vi "main.vi"(11 "launched":refnum<notifier>) -> ()   [LabVIEW 2020]
uses:
  _controls/save_options.ctl
  _controls/checkbox.ctl
  _controls/button.rec.ctl
  camera/camera.lvclass
  <vilib>/Utility/sysdir.llb/System Directory Type.ctl
  _controls/state.ctl
  _controls/DLL.state.ctl
  fb840919-9eb0-46b6-9bb3-d477681bf041.vi
  1d8e8226-7041-439d-8714-8787373e7ba9.vi
  8fbd63eb-6e1f-4c86-bab6-28681c6e18d2.vi
  86724869-5739-4cd7-b902-c7d6e6aa67a1.vi
  55541a10-fe72-4f23-aa32-8552e1fca114.vi
  782ab28e-0829-4b0f-8f82-3ba71064f937.vi
  21b5fd2b-e315-48a8-934d-9fb4121eccaa.vi
  c147b8e2-e97a-4fb6-9f9b-10b3bfa32c03.vi
  d040b064-8120-4bee-ba75-bc9a352b41e4.vi
  f030127b-7363-4f40-9caf-aa7af2fa5467.vi
  a77384f8-0254-4858-83b2-e693f57fe95f.vi
  c0d7e7e1-aa2c-47d6-a73c-058c71d33236.vi
  eef2a813-7c02-4df4-9d88-e87a40ecc536.vi
  96ad7128-a59b-4646-90f0-c775a03dfb8e.vi
  094a7fb3-58c3-48c3-896b-6fa17c1e0ca1.vi
  06917477-7661-483e-91a3-5a2f461782c2.vi
  e584de4e-bacd-4d82-b84f-7ed3eb6609c4.vi
  8bc19d28-31cb-4a7e-a618-0f8835e17850.vi
  3f5928e4-84ec-4848-af44-f012adbf1426.vi
  56f6947d-e80c-43c6-ba91-a3ae61841505.vi
  SubVI/img.Percentile.vi
  SubVI/pix.sgl.CalcPercentiles.sgl.vi
  <vilib>/Utility/file.llb/Application Directory.vi
  <vilib>/Utility/config.llb/Open Config Data.vi
  <vilib>/Utility/config.llb/Read Key.vi
  <vilib>/Utility/config.llb/Read Key (Boolean).vi
  <vilib>/Utility/config.llb/Write Key.vi
  <vilib>/Utility/config.llb/Write Key (Boolean).vi
  SubVI/error.RebrandExistingError.vi
  <vilib>/Utility/config.llb/Close Config Data.vi
  <vilib>/Utility/config.llb/Read Key (String).vi
  <vilib>/Utility/config.llb/Write Key (String).vi
  <vilib>/Utility/config.llb/Read Key (U32).vi
  <vilib>/Utility/config.llb/Write Key (U32).vi
  <vilib>/Utility/config.llb/Read Key (Double).vi
  <vilib>/Utility/config.llb/Write Key (Double).vi
  <vilib>/Utility/config.llb/Read Key (I32).vi
  <vilib>/Utility/config.llb/Write Key (I32).vi
  <vilib>/Utility/config.llb/Read Key (Path).vi
  <vilib>/Utility/config.llb/Write Key (Path).vi
  _accessors/DVR.vars.Read.vi
  SubVI/acq.Filename.vi
  <vilib>/Utility/libraryn.llb/Check if File or Folder Exists.vi
  SubVI/file.IsValid.vi
  SubVI/pix.sgl.CalcPercentiles.vi
  36df9122-e4f2-4645-ba20-61a7cd497c98.vi
panel:
  out "msg":string="Closing Program..."
  in  "fit":bool
  in  "minus":bool
  in  "plus":bool
  in  "FPS (For PL only)":dbl=30.0 min=5.0 max=100.0 step=5.0
  in  "array":bool
  out "recording":string="Recording..."
  in  "Exposure":u32=30 min=5 max=1000 step=5
  out "Image":T1(plugin-control)
  out "sub#":string
  in  "rightTab":enum32{"Acquisition", "Settings"}(tab)
  in  "state":T2(radio)=enum."Video"
  in  "Same?":T3
  in  "#":u32
  in  "video":T4 caption="Save Video"
  in  "histogram.enable":bool caption="Enable"
  in  "# bins":i32=20 caption="Bins bins" min=5 max=50 step=1
  in  "save.op":T5 caption="Save Option"
  in  "base_folder":cluster{"folder":path, "Tif":bool, "Jpg":bool}={"folder"=path "", "Tif"=TRUE, "Jpg"=TRUE}
  in  "Gain":enum16{"Low", "High"}(ring)
  out "histogram":cluster{"Axis":dbl[], "Histogram":i32[]}(graph)
  in  "Acquisitions":u64=5 min=1 max=500 step=1
  in  "Module Name":string="Module"
  in  "Min Value":i32=3 min=0 max=65535
  in  "Max Value":i32=97 min=1 max=65535
  in  "mapping":u32(ring)=16 items=["Default"=10, "Most Significant Bits"=11, "Full Dynamic"=12, "Downshift"=13, "Given Range"=14, "90% Dynamic"=15, "Given Percent Range"=16]
  out "progress":u8(slide) scale=0.0..10.0
  # "ACQ PARAMETERS"
  # "CAMERA"
  # "ACQUISITION"
  # "SAVE"
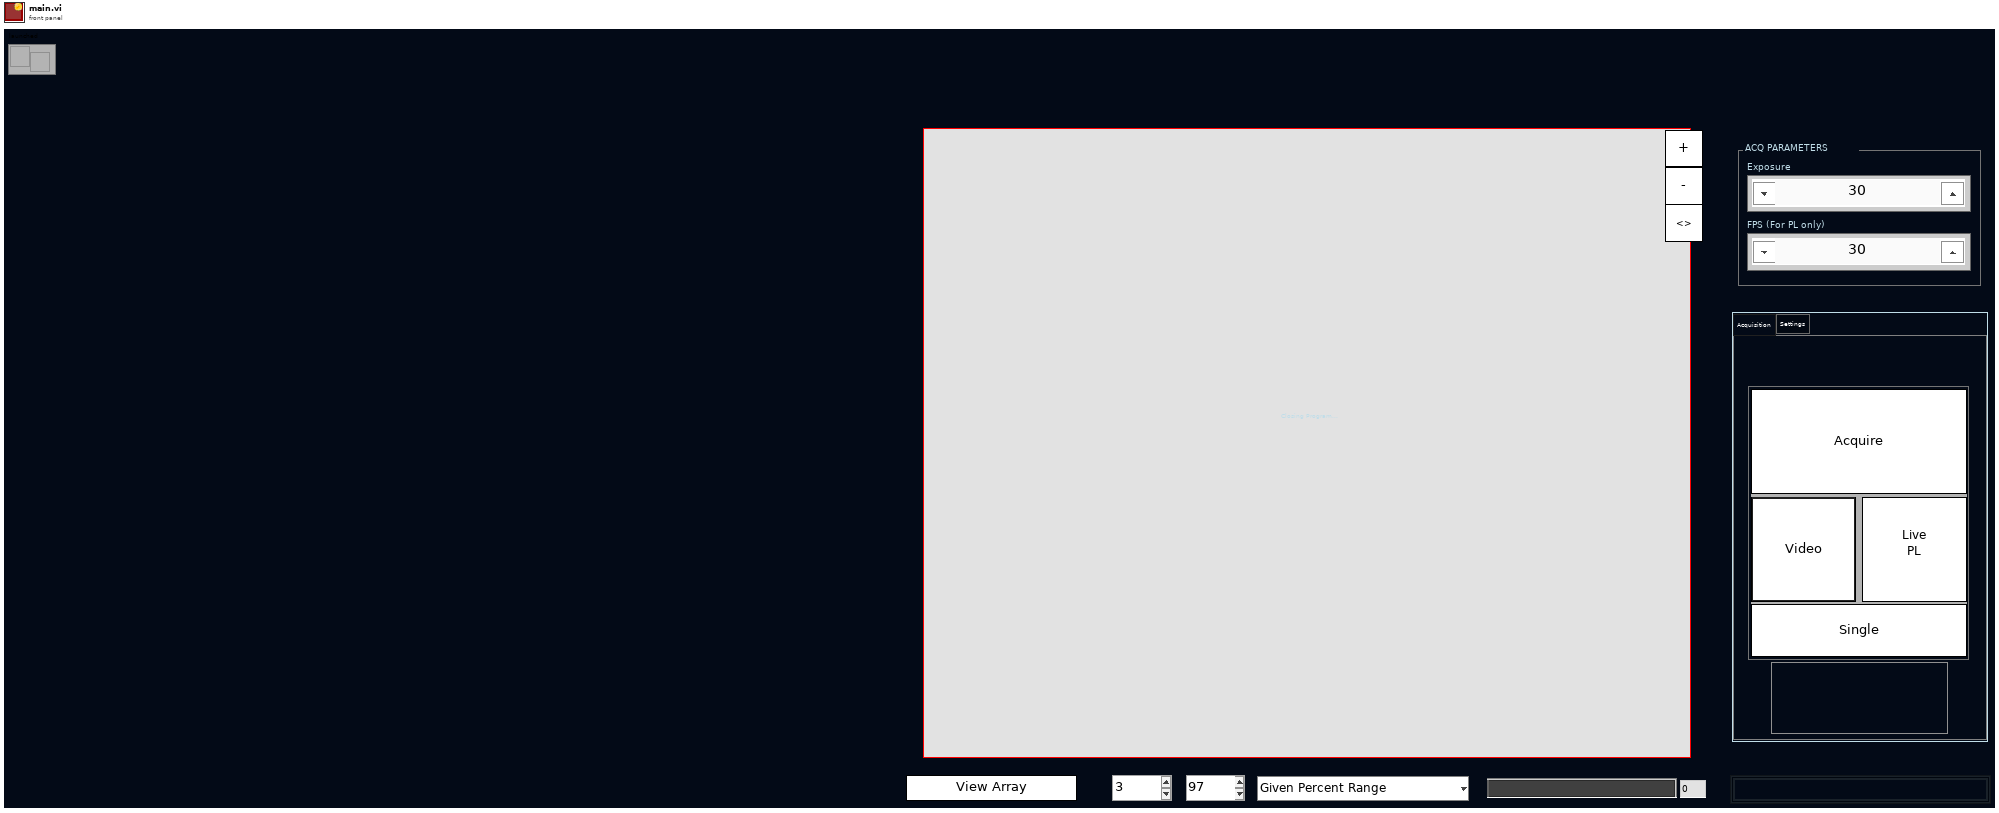
[diagram p1: front panel]
types:
  T1 = typedef "IMAQ Image.ctl" = refnum<image>
  T2 = enum32{"Switch", "Single", "Video", "Live", "none"}
  T3 = typedef "checkbox.ctl" = bool
  T4 = typedef "button.rec.ctl" = bool
  T5 = typedef "save_options.ctl" = enum16{"Light", "Full"}
  T6 = typedef "data.ctl" = cluster{"cam":refnum<class "camera.lvclass">, "ref":T7, "Q":cluster{"acq":cluster{"img1":refnum<queue>}, "display":cluster{"image":refnum<queue>}}, "timing":cluster{"state":refnum<queue>, "closeLoop":refnum<notifier>, "stop":refnum<k4>}, "vars":refnum<data-value>}
  T7 = typedef "data.ref.ctl" = cluster{"This VI":refnum<vi>, "rightPanel":refnum<vi>, "btn":cluster{"action":cluster{"Single":refnum<vi>, "Live":refnum<vi>, "Switch":refnum<vi>, "Video":refnum<vi>}, "Close":refnum<vi>}, "control":cluster{"#":refnum<vi>, "sub#":refnum<vi>, "auto_exp":refnum<vi>, "# Acq":refnum<vi>, "recording":refnum<vi>}, "graph":cluster{"img":T1, "avi":T1}}
  T8 = enum8{"Enabled", "Disabled", "Disabled and Grayed Out"}
  T9 = typedef "state.ctl" = enum16{"-", "single", "video", "livePL", "PL"}
  T10 = cluster{"Left":i32, "Top":i32, "Right":i32, "Bottom":i32}
  T11 = typedef "Image Type" = u32
  T12 = typedef "System Directory Type.ctl" = i32
  T13 = typedef "DLL.state.ctl" = u16
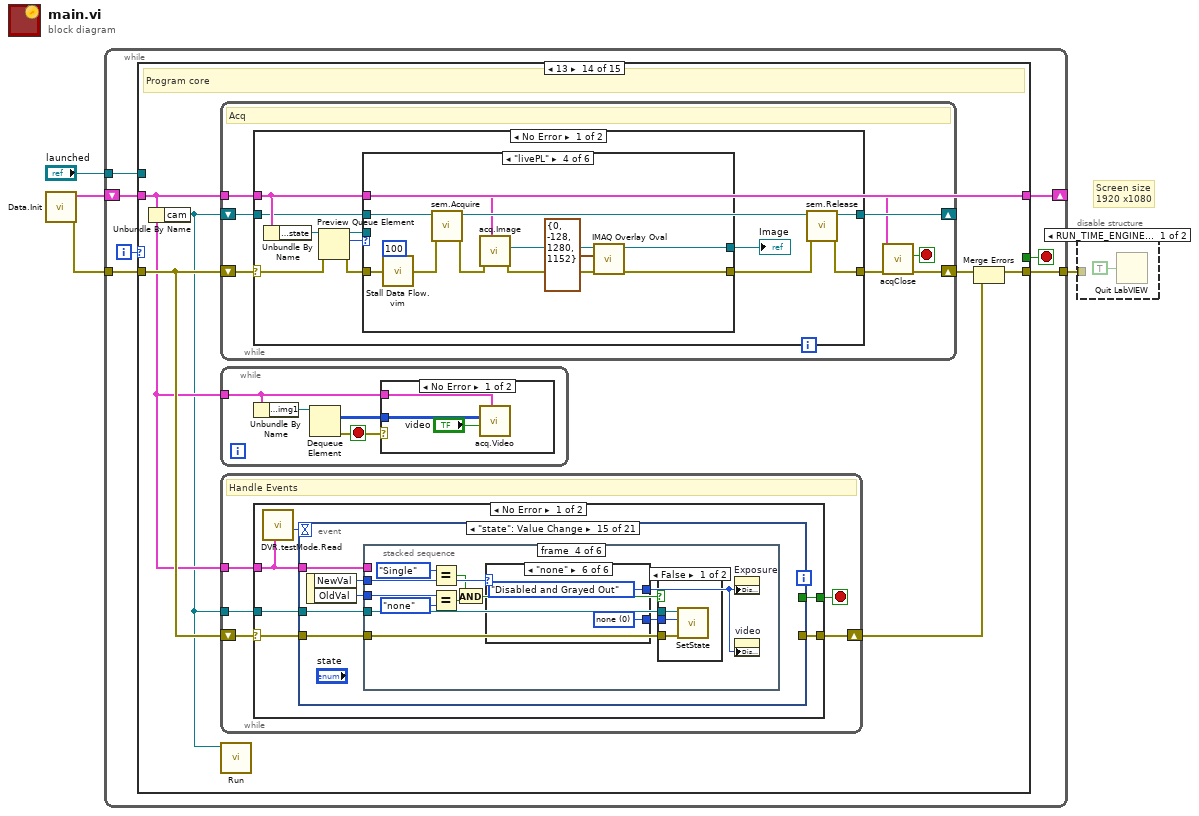
[diagram p0: block diagram]
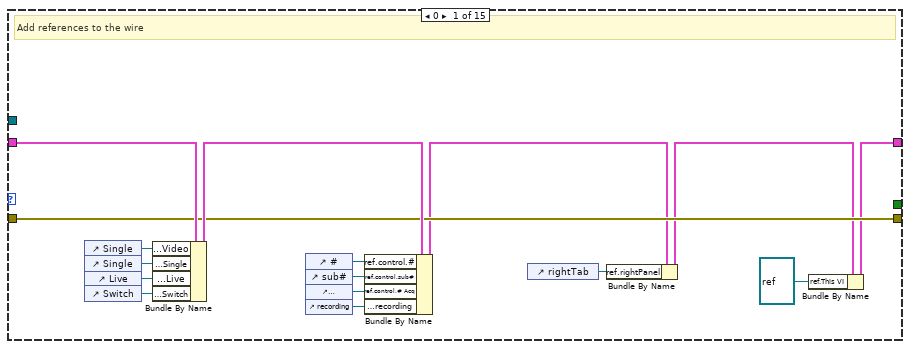
[diagram p2: hidden frame]
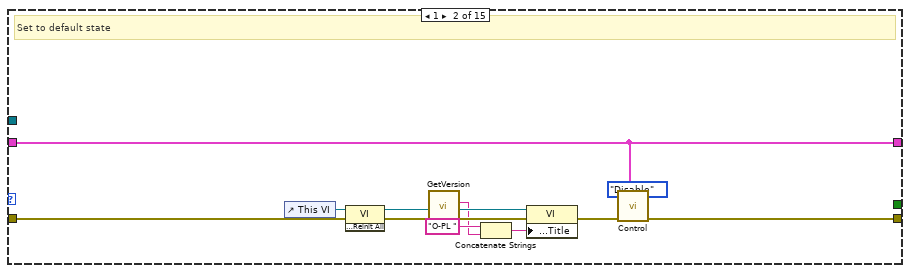
[diagram p3: hidden frame]
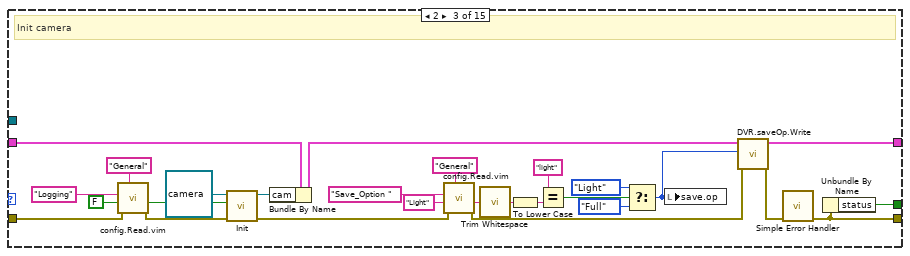
[diagram p4: hidden frame]
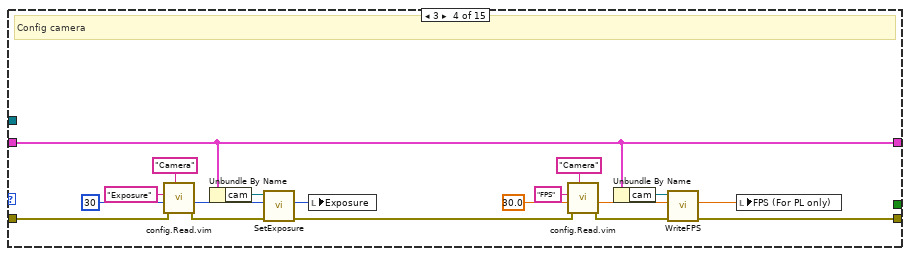
[diagram p5: hidden frame]
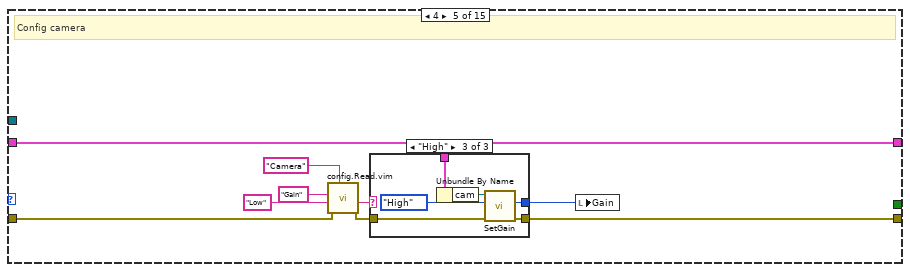
[diagram p6: hidden frame]
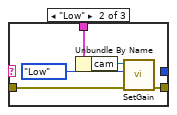
[diagram p8: hidden frame]
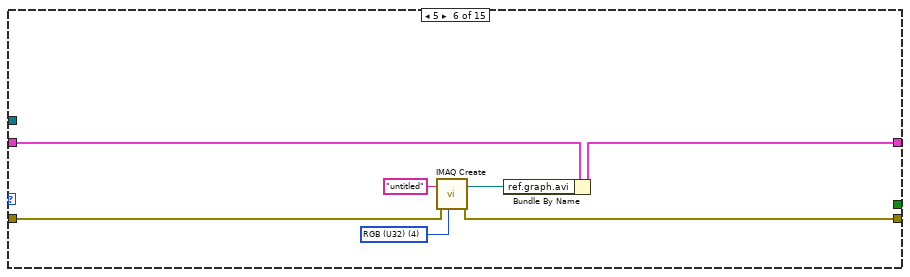
[diagram p9: hidden frame]
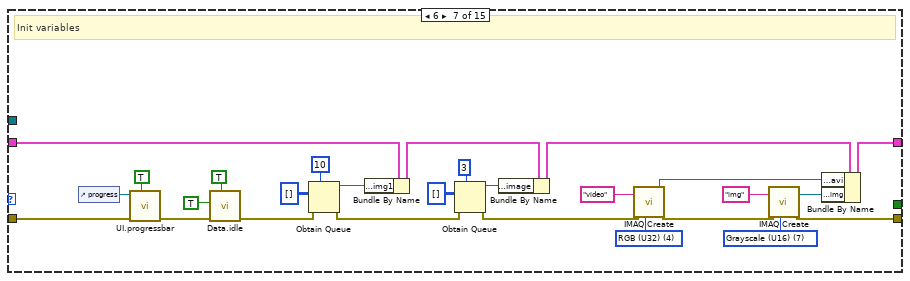
[diagram p10: hidden frame]
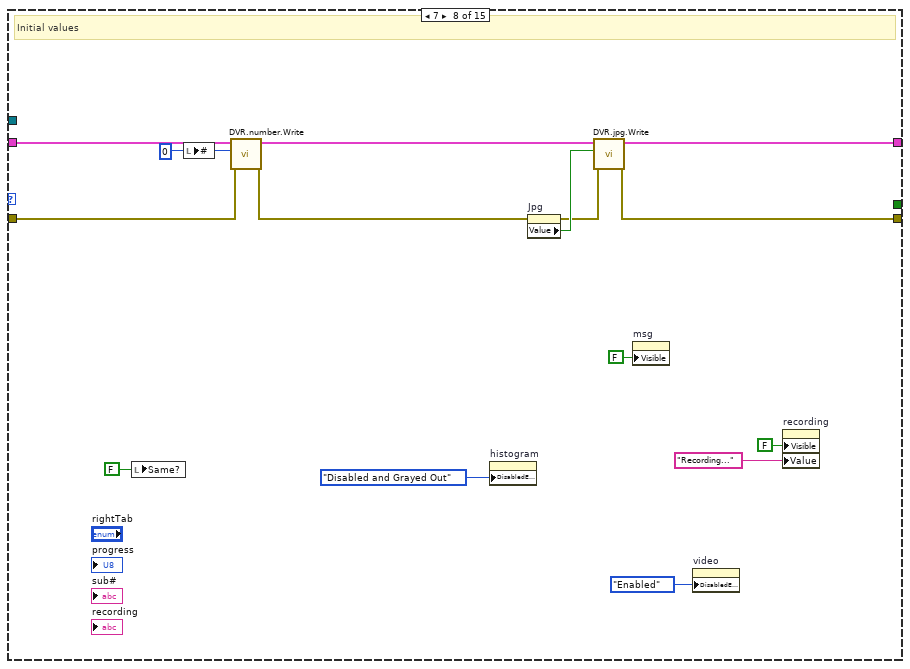
[diagram p11: hidden frame]
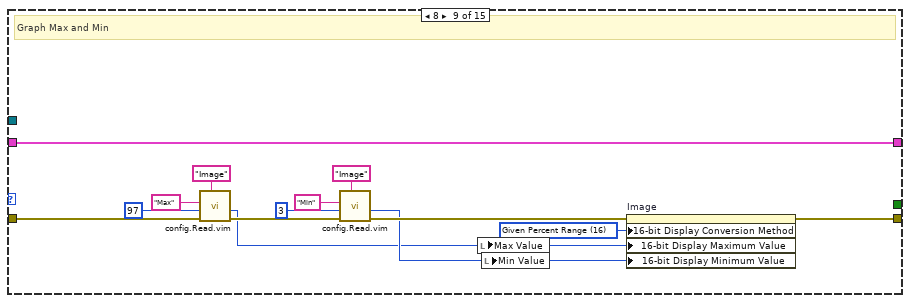
[diagram p12: hidden frame]
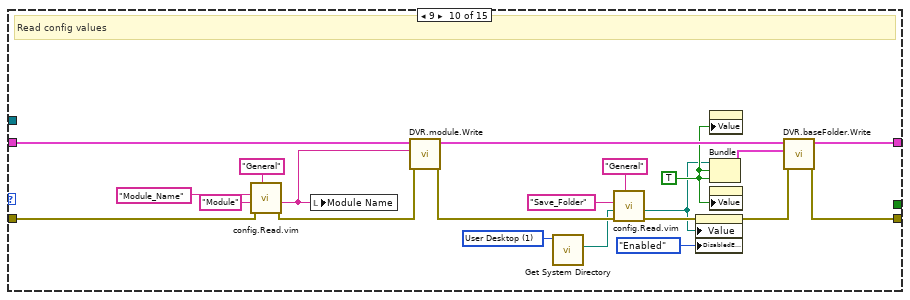
[diagram p13: hidden frame]
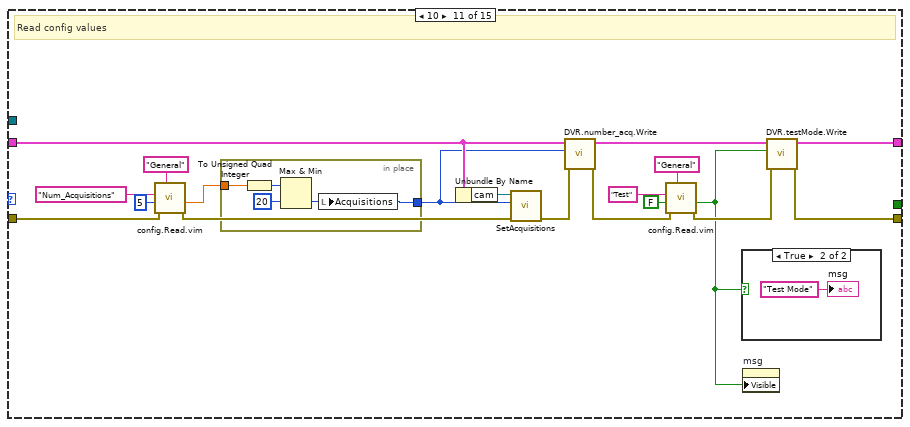
[diagram p14: hidden frame]
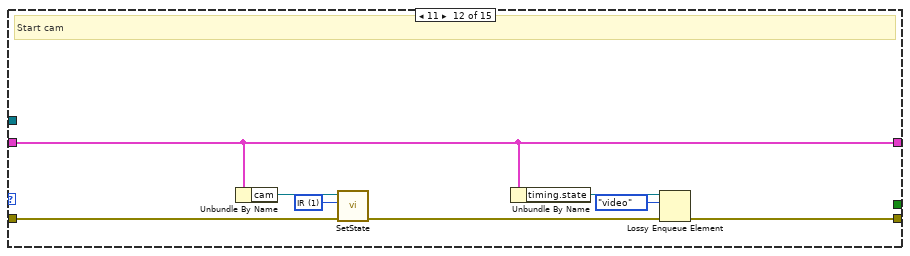
[diagram p16: hidden frame]
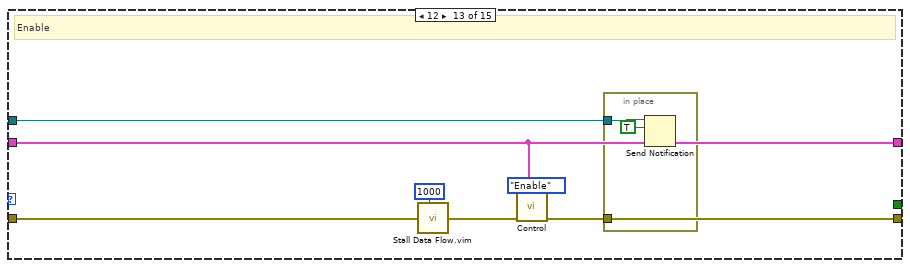
[diagram p17: hidden frame]
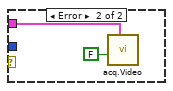
[diagram p18: hidden frame]
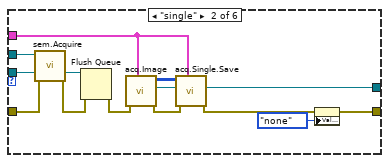
[diagram p20: hidden frame]
diagram:
  # "Screen size\n1920 x1080"
  n1 = call "Data.Init.vi"() -> ("error out"=w2:errorcluster, "DVR"=w4:T6)  [unwired: 10 in]
  n2 = while {
    shift-right: [w6] -> _
    shift-left: w4 -> [w11]
    tunnel: w2 -> [w10]
    tunnel: [w8] -> w3
    tunnel: "launched" -> [w5]
    i -> [w9]
    stop <- w7 stop-if-true
    n3 = case shown="13" w9 {
      tunnel: w11 -> [w27 w37 w65 w67 w89 w105 w132 w142 w149 w179 w186 w207 w216 w222 w514]
      tunnel: w10 -> [w25 w35 w62 w81 w88 w106 w124 w147 w158 w181 w198 w208 w218 w223 w512]
      tunnel: [w25 w38 w63 w66 w90 w102 w120 w145 w161 w180 w184 w211 w213 w225 w516] -> w8
      tunnel: [_ _ w64 _ _ _ _ _ _ _ _ _ _ _ TRUE ("status")] -> w7
      tunnel: [w20 w37 w52 w67 w89 w104 w123 w142 w149 w179 w186 w207 w216 w222 _] -> w6
      tunnel: w5 -> [_ _ _ _ _ _ _ _ _ _ _ _ w212 _ _]
      frame 0 {
        # "Add references to the wire"
        n4 = control-ref of="Single"() -> (w14:refnum<vi>)
        n5 = control-ref of="Single"() -> (w15:refnum<vi>)
        n6 = control-ref of="Live"() -> (w17:refnum<vi>)
        n7 = control-ref of="Switch"() -> (w16:refnum<vi>)
        n8 = Bundle By Name(cluster=w27, "ref.btn.action.Video"=w14, "ref.btn.action.Single"=w15, "ref.btn.action.Live"=w17, "ref.btn.action.Switch"=w16) -> (w26:T6)
        n9 = control-ref of="#"() -> (w24:refnum<vi>)
        n10 = control-ref of="sub#"() -> (w23:refnum<vi>)
        n11 = control-ref of="Acquisitions"() -> (w13:refnum<vi>)
        n12 = control-ref of="recording"() -> (w12:refnum<vi>)
        n13 = Bundle By Name(cluster=w26, "ref.control.#"=w24, "ref.control.sub#"=w23, "ref.control.# Acq"=w13, "ref.control.recording"=w12) -> (w19:T6)
        n14 = control-ref of="rightTab"() -> (w21:refnum<vi>)
        n15 = Bundle By Name(cluster=w19, "ref.rightPanel"=w21) -> (w18:T6)
        n16 = Bundle By Name(cluster=w18, "ref.This VI"=refnum<vi> refnum ("This VI")) -> (w20:T6)
      }
      frame 1 {
        # "Set to default state"
        n17 = control-ref of="This VI"() -> (w36:refnum<vi>)
        n18 = invoke class="VI" method="Default Vals.Reinit All"(reference=w36, error in=w35) -> (reference out=w33:refnum<vi>, error out=w34:errorcluster)  [unwired: 1 in, 1 out]
        n19 = call "GetVersion.vi"("Error In"=w34) -> ("error out"=w32:errorcluster, "Version String"=w29:string)  [unwired: 8 in, 1 out]
        n20 = Concatenate Strings("O-PL ", w29) -> (w28:string)
        n21 = property class="VI"(reference=w33, error in=w32, "Front Panel.Title"=w28) -> (error out=w31:errorcluster)  [unwired: 1 out]
        n22 = call "Control.vi"("mode"=enum16{"Enable", "Disable"}."Disable", "DVR"=w37, "error in"=w31) -> ("error out"=w38:errorcluster)  [unwired: 8 in]
      }
      frame 2 {
        # "Init camera"
        n23 = call "config.Read.vim"("section"="General", "error in"=w62, "default value (F)"=FALSE, "key"="Logging") -> ("error out"=w41:errorcluster, "value out"=w40:bool)  [unwired: 5 in, 1 out]
        n24 = call-dynamic "Init.vi"("error in"=w41, "log?"=w40, "camera.nit in"=refnum<class "camera.lvclass"> refnum ("camera.nit_c.lvclass")) -> ("error out"=w59:errorcluster, "camera.nit out"=w46:refnum<class "camera.lvclass">)  [unwired: 7 in]
        n25 = Bundle By Name(cluster=w65, "cam"=w46) -> (w52:T6)
        n26 = call "config.Read.vim"("section"="General", "error in"=w59, "default value (F)"="Light", "key"="Save_Option ") -> ("error out"=w48:errorcluster, "value out"=w57:string)  [unwired: 5 in, 1 out]
        n27 = call <vilib>:"Trim Whitespace.vi"("string"=w57) -> ("trimmed string"=w55:string)  [unwired: 1 in]
        n28 = To Lower Case(string=w55) -> (all lower case string=w54:string)
        n29 = Equal?(x="light", y=w54) -> (x = y?=w53:bool)
        n30 = Select(t=save_options."Light" ("save.op"), s=w53, f=save_options."Full") -> (s? t:f=w49:T5)
        n31 = local write "save.op"(w49) -> ()
        n32 = call "DVR.saveOp.Write.vi"("error in"=w48, "save.save.op"=w49, "DVR in"=w52) -> ("error out"=w47:errorcluster)  [unwired: 8 in]
        n33 = call <vilib>:"Simple Error Handler.vi"("error in (no error)"=w47) -> ("error out"=w63:errorcluster)  [unwired: 4 in, 4 out]
        n34 = Unbundle By Name(w63) -> ("status"=w64:bool)
      }
      frame 3 {
        # "Config camera"
        n35 = call "config.Read.vim"("section"="Camera", "error in"=w81, "default value (F)"=u32 30 ("Exp"), "key"="Exposure") -> ("error out"=w77:errorcluster, "value out"=w75:u32)  [unwired: 5 in, 1 out]
        n36 = Unbundle By Name(w67) -> ("cam"=w76:refnum<class "camera.lvclass">)
        n37 = call-dynamic "SetExposure.vi"("error in"=w77, "Exp"=w75, "camera.nit in"=w76) -> ("error out"=w68:errorcluster)  [unwired: 8 in]
        n38 = local write "Exposure"(w75) -> ()
        n39 = call "config.Read.vim"("section"="Camera", "error in"=w68, "default value (F)"=30.0 ("Exp"), "key"="FPS") -> ("error out"=w72:errorcluster, "value out"=w74:dbl)  [unwired: 5 in, 1 out]
        n40 = Unbundle By Name(w67) -> ("cam"=w73:refnum<class "camera.lvclass">)
        n41 = call-dynamic "WriteFPS.vi"("error in"=w72, "FPS"=w74, "camera.nit in"=w73) -> ("error out"=w66:errorcluster)  [unwired: 8 in]
        n42 = local write "FPS (For PL only)"(w74) -> ()
      }
      frame 4 {
        # "Config camera"
        n43 = call "config.Read.vim"("section"="Camera", "error in"=w88, "default value (F)"="Low" ("key"), "key"="Gain") -> ("error out"=w84:errorcluster, "value out"=w82:string)  [unwired: 5 in, 1 out]
        n44 = case shown="\"High\"" w82 {
          tunnel: w84 -> [w91 w96 w101]
          tunnel: [w91 w95 w100] -> w90
          tunnel: w89 -> [_ w93 w99]
          tunnel: [_ _ w97] -> w87
          frame Default {
          }
          frame "Low" {
            n45 = Unbundle By Name(w93) -> ("cam"=w92:refnum<class "camera.lvclass">)
            n46 = call "SetGain.vi"("error in"=w96, "Gain"=enum16{"Low", "High"}."Low", "camera.nit in"=w92) -> ("error out"=w95:errorcluster)  [unwired: 8 in]
          }
          frame "High" {
            w97 = enum16{"Low", "High"}."High" ("Gain")
            n47 = Unbundle By Name(w99) -> ("cam"=w98:refnum<class "camera.lvclass">)
            n48 = call "SetGain.vi"("error in"=w101, "Gain"=w97, "camera.nit in"=w98) -> ("error out"=w100:errorcluster)  [unwired: 8 in]
          }
        }
        n49 = local write "Gain"(w87) -> ()
      }
      frame 5 {
        w108 = T11 4 items=["Grayscale (U8)", "Grayscale (I16)", "Grayscale (SGL)", "Complex (CSG)", "RGB (U32)", "HSL (U32)", "RGB (U64)", "Grayscale (U16)"] ("Image Type")
        n50 = call "IMAQ Create"("Image Name"="untitled", "Image Type"=w108, "error in (no error)"=w106) -> ("New Image"=w103:T1, "error out"=w102:errorcluster)  [unwired: 2 in]
        n51 = Bundle By Name(cluster=w105, "ref.graph.avi"=w103) -> (w104:T6)
      }
      frame 6 {
        w116 = T11 4 items=["Grayscale (U8)", "Grayscale (I16)", "Grayscale (SGL)", "Complex (CSG)", "RGB (U32)", "HSL (U32)", "RGB (U64)", "Grayscale (U16)"] ("Image Type")
        w122 = T11 7 items=["Grayscale (U8)", "Grayscale (I16)", "Grayscale (SGL)", "Complex (CSG)", "RGB (U32)", "HSL (U32)", "RGB (U64)", "Grayscale (U16)"] ("Image Type")
        # "Init variables"
        n52 = control-ref of="progress"() -> (w135:refnum<vi>)
        n53 = call "UI.progressbar.vi"("write?"=TRUE, "error in"=w124, "Slide in"=w135) -> ("error out"=w133:errorcluster)  [unwired: 8 in]
        n54 = call "Data.idle.vi"("write?"=TRUE, "error in"=w133, "idle in"=TRUE) -> ("error thru"=w111:errorcluster)  [unwired: 7 in, 1 out]
        n55 = Obtain Queue(max queue size (-1, unlimited)=10, element data type=u16[][] [] ("buffer"), error in (no error)=w111) -> (queue out=w129:refnum<queue>, error out=w110:errorcluster)  [unwired: 2 in, 1 out]
        n56 = Bundle By Name(cluster=w132, "Q.acq.img1"=w129) -> (w118:T6)
        n57 = Obtain Queue(max queue size (-1, unlimited)=3, element data type=u16[][] [] ("buffer"), error in (no error)=w110) -> (queue out=w128:refnum<queue>, error out=w109:errorcluster)  [unwired: 2 in, 1 out]
        n58 = Bundle By Name(cluster=w118, "Q.display.image"=w128) -> (w125:T6)
        n59 = call "IMAQ Create"("Image Name"="video", "Image Type"=w116, "error in (no error)"=w109) -> ("New Image"=w115:T1, "error out"=w114:errorcluster)  [unwired: 2 in]
        n60 = call "IMAQ Create"("Image Name"="img", "Image Type"=w122, "error in (no error)"=w114) -> ("New Image"=w119:T1, "error out"=w120:errorcluster)  [unwired: 2 in]
        n61 = Bundle By Name(cluster=w125, "ref.graph.avi"=w115, "ref.graph.img"=w119) -> (w123:T6)
      }
      frame 7 {
        w148 = 0 ("#")
        # "Initial values"
        n62 = local write "Same?"(FALSE ("same?")) -> ()
        n63 = local write "#"(w148) -> ()
        n64 = call "DVR.number.Write.vi"("error in"=w147, "save.#"=w148, "DVR in"=w142) -> ("error out"=w137:errorcluster)  [unwired: 8 in]
        n65 = property on="histogram" class="XYGraph (strict)"("DisabledEnum"=T8."Disabled and Grayed Out" ("Disabled")) -> ()  [unwired: 2 in, 2 out]
        n66 = property on="Jpg" class="Bool (strict)"(error in=w137) -> (error out=w143:errorcluster, "Value"=w144:bool)  [unwired: 1 in, 1 out]
        n67 = call "DVR.jpg.Write.vi"("error in"=w143, "jpg?"=w144, "DVR in"=w142) -> ("error out"=w145:errorcluster)  [unwired: 8 in]
        n68 = property on="msg" class="Str"("Visible"=FALSE) -> ()  [unwired: 2 in, 2 out]
        n69 = property on="video" class="Bool (strict)"("DisabledEnum"=T8."Enabled" ("Disabled")) -> ()  [unwired: 2 in, 2 out]
        n70 = property on="recording" class="Str"("Visible"=FALSE, "Value"="Recording..." ("recording")) -> ()  [unwired: 2 in, 2 out]
      }
      frame 8 {
        w162 = u32 16 items=["Default"=10, "Most Significant Bits"=11, "Full Dynamic"=12, "Downshift"=13, "Given Range"=14, "90% Dynamic"=15, "Given Percent Range"=16] ("16-bit Display Mapping:Conversion Method")
        # "Graph Max and Min"
        n71 = call "config.Read.vim"("section"="Image", "error in"=w158, "default value (F)"=97 ("16-bit Display Mapping:Maximum Value"), "key"="Max") -> ("error out"=w155:errorcluster, "value out"=w150:i32)  [unwired: 5 in, 1 out]
        n72 = call "config.Read.vim"("section"="Image", "error in"=w155, "default value (F)"=3 ("16-bit Display Mapping:Minimum Value"), "key"="Min") -> ("error out"=w154:errorcluster, "value out"=w151:i32)  [unwired: 5 in, 1 out]
        n73 = local write "Max Value"(w150) -> ()
        n74 = local write "Min Value"(w151) -> ()
        n75 = property on="Image" class="ImageControl"(error in=w154, "16-bit Display Conversion Method"=w162, "16-bit Display Maximum Value"=w150, "16-bit Display Minimum Value"=w151) -> (error out=w161:errorcluster)  [unwired: 1 in, 1 out]
      }
      frame 9 {
        w172 = T12 1 items=["User Home"=0, "User Desktop"=1, "User Documents"=2, "User Application Data"=3, "User Preferences"=4, "User Temporary"=5, "Public Documents"=6, "Public Application Data"=7, "Public Preferences"=8, "Public Cache"=13, "System Core Libraries"=9, "System Installed Libraries"=10, "Application Files"=11, "Boot Volume Root"=12] ("system directory type")
        w169 = TRUE
        # "Read config values"
        n76 = call "config.Read.vim"("section"="General", "error in"=w181, "default value (F)"="Module", "key"="Module_Name") -> ("error out"=w164:errorcluster, "value out"=w163:string)  [unwired: 5 in, 1 out]
        n77 = local write "Module Name"(w163) -> ()
        n78 = call "DVR.module.Write.vi"("error in"=w164, "module"=w163, "DVR in"=w179) -> ("error out"=w178:errorcluster)  [unwired: 8 in]
        n79 = call <vilib>:"Get System Directory.vi"("system directory type"=w172) -> ("system directory"=w171:path)  [unwired: 10 in]
        n80 = call "config.Read.vim"("section"="General", "error in"=w178, "default value (F)"=w171, "key"="Save_Folder") -> ("error out"=w173:errorcluster, "value out"=w168:path)  [unwired: 5 in, 1 out]
        n81 = property on="folder" class="Path"(error in=w173, "Value"=w168, "DisabledEnum"=T8."Enabled" ("Disabled")) -> (error out=w165:errorcluster)  [unwired: 1 in, 1 out]
        n82 = property on="Tif" class="Bool (strict)"("Value"=w169) -> ()  [unwired: 2 in, 2 out]
        n83 = Bundle("value out"=w168, w169, w169) -> (w170:cluster{"value out":path, bool, bool})  [unwired: 1 in]
        n84 = property on="Jpg" class="Bool (strict)"("Value"=w169) -> ()  [unwired: 2 in, 2 out]
        n85 = call "DVR.baseFolder.Write.vi"("error in"=w165, "save.base_folder"=w170, "DVR in"=w179) -> ("error out"=w180:errorcluster)  [unwired: 8 in]
      }
      frame 10 {
        # "Read config values"
        n86 = call "config.Read.vim"("section"="General", "error in"=w198, "default value (F)"=u64 5 ("# Acq"), "key"="Num_Acquisitions") -> ("error out"=w195:errorcluster, "value out"=w192:dbl)  [unwired: 5 in, 1 out]
        n87 = in-place {
          in-place-border: w192 -> [w203]
          in-place-border: [w200] -> w183
          n88 = To Unsigned Quad Integer(1:w203) -> (0:w202:u64)
          n89 = Max & Min(x=w202, y=u64 20 ("x")) -> (min(x,y)=w200:u64)  [unwired: 1 out]
          n90 = local write "Acquisitions"(w200) -> ()
        }
        n91 = Unbundle By Name(w186) -> ("cam"=w197:refnum<class "camera.lvclass">)
        n92 = call "SetAcquisitions.vi"("error in"=w195, "Acquisitions"=w183, "camera in"=w197) -> ("error out"=w191:errorcluster)  [unwired: 8 in]
        n93 = call "DVR.number_acq.Write.vi"("error in"=w191, "# acq"=w183, "DVR in"=w186) -> ("error out"=w187:errorcluster)  [unwired: 8 in]
        n94 = call "config.Read.vim"("section"="General", "error in"=w187, "default value (F)"=FALSE, "key"="Test") -> ("error out"=w185:errorcluster, "value out"=w182:bool)  [unwired: 5 in, 1 out]
        n95 = case shown="True" w182 {
          frame False {
          }
          frame True {
            "msg" <- "Test Mode" ("msg")
          }
        }
        n96 = property on="msg" class="Str"("Visible"=w182) -> ()  [unwired: 2 in, 2 out]
        n97 = call "DVR.testMode.Write.vi"("error in"=w185, "Test Mode"=w182, "DVR in"=w186) -> ("error out"=w184:errorcluster)  [unwired: 8 in]
      }
      frame 11 {
        w205 = T13 1 items=["none", "IR", "PL"] ("DLL.state")
        # "Start cam"
        n98 = Unbundle By Name(w207) -> ("cam"=w204:refnum<class "camera.lvclass">)
        n99 = call "SetState.vi"("error in"=w208, "DLL.state"=w205, "camera in"=w204) -> ("error out"=w209:errorcluster)  [unwired: 8 in]
        n100 = Unbundle By Name(w207) -> ("timing.state"=w210:refnum<queue>)
        n101 = Lossy Enqueue Element(queue=w210, element=state."video", error in (no error)=w209) -> (error out=w211:errorcluster)  [unwired: 3 out]
      }
      frame 12 {
        # "Enable"
        n102 = call "Stall Data Flow.vim"("value in"=w218, "milliseconds to wait"=u32 1000) -> ("value out"=w215:errorcluster)  [unwired: 1 out]
        n103 = call "Control.vi"("mode"=enum16{"Enable", "Disable"}."Enable", "DVR"=w216, "error in"=w215) -> ("error out"=w213:errorcluster)  [unwired: 8 in]
        n104 = in-place {
          in-place-border: w213 -> [_]
          in-place-border: w212 -> [w220]
          n105 = Send Notification(notification=TRUE, notifier=w220) -> ()  [unwired: 1 in, 2 out]
        }
      }
      frame 13 {
        # "Program core"
        n106 = Unbundle By Name(w222) -> ("cam"=w221:refnum<class "camera.lvclass">)
        n107 = while {
          shift-right: [w237] -> w226
          shift-left: w223 -> [w241]
          tunnel: w222 -> [w239]
          shift-right: [w240] -> _
          shift-left: w221 -> [w242]
          stop <- w236 stop-if-true
          # "Acq"
          n108 = case shown="No Error" w241 {
            selector: w241 -> [w249 w302]
            tunnel: [w244 _] -> w238
            tunnel: w242 -> [w245 w303]
            tunnel: w239 -> [w252 _]
            tunnel: [w245 w303] -> w240
            frame No Error {
              n109 = Unbundle By Name(w252) -> ("timing.state"=w251:refnum<queue>)
              n110 = Preview Queue Element(queue=w251, error in (no error)=w249) -> (queue out=w247:refnum<queue>, element=w250:T9, error out=w248:errorcluster)  [unwired: 1 in, 1 out]
              n111 = case shown="\"livePL\"" w250 {
                tunnel: w245 -> [_ w259 w268 w277 w288 w301]
                tunnel: [w253 w260 w269 w278 w289 w300] -> w243
                tunnel: w248 -> [w253 w257 w271 w282 w295 w299]
                tunnel: w252 -> [_ w254 w273 w284 w292 _]
                tunnel: w247 -> [_ w265 _ _ w298 _]
                tunnel: [_ w263 w270 w280 w291 _] -> w246
                frame Default {
                }
                frame "single" {
                  n112 = call "sem.Acquire.vi"("error in"=w257, "camera.nit in"=w259) -> ("error out"=w258:errorcluster)  [unwired: 9 in]
                  n113 = Flush Queue(queue=w265, error in (no error)=w258) -> (error out=w264:errorcluster)  [unwired: 2 out]
                  n114 = call "acq.Image.vi"("DVR"=w254, "error in"=w264) -> ("error out"=w261:errorcluster, "Image Out"=w263:T1, "buffer"=w256:u16[][])  [unwired: 7 in]
                  n115 = call "acq.Single.Save.vi"("DVR"=w254, "error in"=w261, "buffer in"=w256) -> ("error out"=w255:errorcluster)  [unwired: 8 in]
                  n116 = property on="state" class="RadioBtnsControl (strict)"(error in=w255, "Value"=T2."none" ("state")) -> (error out=w260:errorcluster)  [unwired: 1 in, 1 out]
                }
                frame "video" {
                  n117 = call "Stall Data Flow.vim"("value in"=w271, "milliseconds to wait"=u32 100) -> ("value out"=w267:errorcluster)  [unwired: 1 out]
                  n118 = call "sem.Acquire.vi"("error in"=w267, "camera.nit in"=w268) -> ("error out"=w266:errorcluster)  [unwired: 9 in]
                  n119 = call "acq.Image.vi"("DVR"=w273, "error in"=w266) -> ("error out"=w269:errorcluster, "Image Out"=w270:T1)  [unwired: 7 in, 1 out]
                }
                frame "livePL" {
                  n120 = call "Stall Data Flow.vim"("value in"=w282, "milliseconds to wait"=u32 100) -> ("value out"=w276:errorcluster)  [unwired: 1 out]
                  n121 = call "sem.Acquire.vi"("error in"=w276, "camera.nit in"=w277) -> ("error out"=w275:errorcluster)  [unwired: 9 in]
                  n122 = call "acq.Image.vi"("DVR"=w284, "error in"=w275) -> ("error out"=w279:errorcluster, "Image Out"=w281:T1)  [unwired: 7 in, 1 out]
                  n123 = call "IMAQ Overlay Oval"("error in (no error)"=w279, "Bounding Rectangle"=T10 {"Left"=0, "Top"=-128, "Right"=1280, "Bottom"=1152} ("Rectangle"), "Image"=w281) -> ("error out"=w278:errorcluster, "Image Out"=w280:T1)  [unwired: 7 in]
                }
                frame "PL" {
                  (unwired) TRUE ("updateGraph")
                  n124 = call "sem.Acquire.vi"("error in"=w295, "camera.nit in"=w288) -> ("error out"=w296:errorcluster)  [unwired: 9 in]
                  n125 = Flush Queue(queue=w298, error in (no error)=w296) -> (error out=w297:errorcluster)  [unwired: 2 out]
                  n126 = local read "Max Value"() -> (w286:i32)
                  n127 = local read "Min Value"() -> (w285:i32)
                  n128 = call "acq.PL.vi"("DVR"=w292, "error in"=w297) -> ("error out"=w293:errorcluster, "Refnum out"=w291:T1, "buffer"=w294:u16[][])  [unwired: 7 in]
                  n129 = call "module.Layouts.vi"("Min Value"=w285, "camera.nit in"=w288, "Max Value"=w286, "DVR"=w292, "error in"=w293, "Image"=w291, "buffer"=w294) -> ("error out"=w287:errorcluster)  [unwired: 4 in]
                  n130 = property on="Live" class="Bool (strict)"(error in=w287, "Val(Sgnl)"=TRUE ("Value (Signaling)")) -> (error out=w289:errorcluster)  [unwired: 1 in, 1 out]
                }
                frame "-" {
                  n131 = call "sem.Acquire.vi"("error in"=w299, "camera.nit in"=w301) -> ("error out"=w300:errorcluster)  [unwired: 9 in]
                }
              }
              "Image" <- w246
              n132 = call "sem.Release.vi"("error in"=w243, "camera.nit in"=w245) -> ("error out"=w244:errorcluster)  [unwired: 9 in]
            }
            frame Error {
              n133 = call <vilib>:"Simple Error Handler.vi"("error in (no error)"=w302) -> ()  [unwired: 4 in, 5 out]
            }
          }
          n134 = call "acqClose.vi"("error in"=w238, "DVR in"=w239) -> ("error out"=w237:errorcluster, "close?"=w236:bool)  [unwired: 8 in]
        }
        n135 = while {
          tunnel: w222 -> [w227]
          stop <- w229 stop-if-true
          n136 = Unbundle By Name(w227) -> ("Q.acq.img1"=w230:refnum<queue>)
          n137 = Dequeue Element(queue=w230) -> (element=w228:u16[][], error out=w229:errorcluster)  [unwired: 2 in, 2 out]
          n138 = case shown="No Error" w229 {
            tunnel: w228 -> [w233 _]
            tunnel: w227 -> [w232 w235]
            frame No Error {
              n139 = call "acq.Video.vi"("DVR"=w232, "video"="video", "buffer in"=w233) -> ()  [unwired: 7 in, 2 out]
            }
            frame Error {
              n140 = call "acq.Video.vi"("DVR"=w235, "video"=T3 FALSE) -> ()  [unwired: 8 in, 2 out]
            }
          }
        }
        n141 = while {
          tunnel: w221 -> [w307]
          tunnel: w222 -> [w304]
          shift-right: [w306] -> w224
          shift-left: w223 -> [w305]
          stop <- w308 stop-if-true
          # "Handle Events"
          n142 = case shown="No Error" w305 {
            selector: w305 -> [w311 w511]
            tunnel: [w314 _] -> w308
            tunnel: w307 -> [w313 _]
            tunnel: w304 -> [w309 _]
            tunnel: [w312 _] -> w306
            frame No Error {
              n143 = call "DVR.testMode.Read.vi"("DVR in"=w309) -> ("timeout"=w310:i32)  [unwired: 10 in]
              n144 = event shown="[14] \"state\": Value Change" {
                selector: _ -> [_ _ _ _ _ _ _ _ _ _ _ _ _ _ _ _ _ _ _ _ _]
                dyn-events: _ -> [_ _ _ _ _ _ _ _ _ _ _ _ _ _ _ _ _ _ _ _ _]
                timeout: w310 -> [_ _ _ _ _ _ _ _ _ _ _ _ _ _ _ _ _ _ _ _ _]
                tunnel: [_ _ w333 w337 w340 w347 w348 w352 w364 w370 w385 w401 _ _ _ _ _ w486 w492 w500 w510] -> w312
                tunnel: [TRUE ("notification") _ _ _ _ _ _ _ _ _ _ _ _ _ _ _ _ _ _ _ _] -> w314
                tunnel: w313 -> [_ _ _ _ _ _ _ _ _ w368 w383 w402 _ _ w416 _ w479 w490 _ _ _]
                tunnel: w309 -> [w321 _ w335 w338 w341 w346 w349 w356 w365 w369 w384 _ _ _ w419 _ _ w489 _ _ _]
                tunnel: w311 -> [_ _ _ _ _ _ _ w351 w363 w371 w386 _ _ _ w418 _ _ w491 w497 w505 w509]
                event Panel Close? {
                  w317 = T3 FALSE ("video")
                  n145 = event-data() -> ()  [unwired: 1 in, 1 out]
                  n146 = local write "video"(w317) -> ()
                  n147 = in-place {
                    in-place-border: w321 -> [w324]
                    in-place-border: w317 -> [w323]
                    in-place-border: [w323] -> w318
                    n148 = call "acq.Stop.vi"("DVR"=w324) -> ()  [unwired: 10 in]
                  }
                  n149 = property on="msg" class="Str"("Value"="Closing Program..." ("closing_msg"), "Visible"=TRUE) -> ()  [unwired: 2 in, 2 out]
                  n150 = call "Stall Data Flow.vim"("value in"=w318, "milliseconds to wait"=u32 100) -> ()  [unwired: 2 out]
                  n151 = event-data("Discard?"=TRUE) -> ()  [unwired: 1 in, 1 out]
                }
                event Timeout {
                  n152 = event-data() -> ()  [unwired: 1 in, 1 out]
                  n153 = feedback #1(u64 0) -> (w325:u64)
                  n154 = Increment(x=w325) -> (x+1=w328:u64)
                  n155 = feedback-in #1(w328) -> ()
                  n156 = Quotient & Remainder(x=w325, y=u64 3) -> (x-y*floor(x/y)=w326:u64)  [unwired: 1 out]
                  n157 = case shown="1" w326 {
                    frame 2, Default {
                      n158 = property on="Video" class="Bool (strict)"("Val(Sgnl)"=TRUE ("Value (Signaling)")) -> ()  [unwired: 2 in, 2 out]
                    }
                    frame 0 {
                      n159 = property on="Live" class="Bool (strict)"("Val(Sgnl)"=TRUE ("Value (Signaling)")) -> ()  [unwired: 2 in, 2 out]
                    }
                    frame 1 {
                      n160 = property on="Switch" class="Bool (strict)"("Val(Sgnl)"=TRUE ("Value (Signaling)")) -> ()  [unwired: 2 in, 2 out]
                    }
                  }
                }
                event Value Change {
                  n161 = event-data() -> ()  [unwired: 1 in, 1 out]
                  n162 = call "DVR.same.Write.vi"("save.same?"="Same?", "DVR in"=w335) -> ("error out"=w333:errorcluster)  [unwired: 9 in]
                }
                event "#": Value Change {
                  n163 = event-data() -> ()  [unwired: 1 in, 1 out]
                  n164 = call "DVR.number.Write.vi"("save.#"="#", "DVR in"=w338) -> ("error out"=w337:errorcluster)  [unwired: 9 in]
                }
                event "base_folder.Jpg": Value Change {
                  n165 = event-data() -> ("NewVal"=w339:bool)  [unwired: 1 in]
                  n166 = call "DVR.jpg.Write.vi"("jpg?"=w339, "DVR in"=w341) -> ("error out"=w340:errorcluster)  [unwired: 9 in]
                }
                event Value Change {
                  n167 = event-data() -> ()  [unwired: 1 in, 1 out]
                  n168 = call "DVR.saveOp.Write.vi"("save.save.op"="save.op", "DVR in"=w346) -> ("error out"=w347:errorcluster)  [unwired: 9 in]
                  n169 = Format Into String("save.op") -> (resulting string=w342:string)  [unwired: 3 in, 1 out]
                  n170 = call "config.Write.vi"("section"="General", "value"=w342, "key"="Save_Option ") -> ()  [unwired: 8 in, 1 out]
                }
                event "array": Value Change {
                  n171 = event-data() -> ()  [unwired: 1 in, 1 out]
                  n172 = call "module.Layouts.Lite.vi"("DVR"=w349) -> ("error out"=w348:errorcluster)  [unwired: 10 in]
                }
                event "base_folder": Value Change {
                  n173 = event-data() -> ()  [unwired: 1 in, 3 out]
                  n174 = call "DVR.baseFolder.Write.vi"("error in"=w351, "save.base_folder"="base_folder", "DVR in"=w356) -> ("error out"=w350:errorcluster)  [unwired: 8 in]
                  n175 = Unbundle By Name("base_folder") -> ("Tif"=w355:bool)
                  n176 = call "conv.Disabled.vi"("NewVal"=w355) -> ("f"=w354:T8)  [unwired: 10 in]
                  n177 = property on="folder" class="Path"(error in=w350, "DisabledEnum"=w354) -> (error out=w352:errorcluster)  [unwired: 1 in, 1 out]
                }
                event "Module Name": Value Change {
                  n178 = event-data() -> ()  [unwired: 1 in, 1 out]
                  n179 = call "string.RemoveIllegalChars.vi"("mode (file)"=enum16{"filename", "database", "alphanumeric"}."filename", "string in"="Module Name") -> ("legal string out"=w360:string)  [unwired: 7 in, 2 out]
                  n180 = String Subset(string=w360, length (rest)=20 ("length (rest)")) -> (substring=w358:string)  [unwired: 1 in]
                  n181 = call "config.Write.vi"("section"="General", "error in"=w363, "value"=w358, "key"="Module_Name") -> ("error out"=w357:errorcluster)  [unwired: 7 in]
                  n182 = local write "Module Name"(w358) -> ()
                  n183 = call "DVR.module.Write.vi"("error in"=w357, "module"=w358, "DVR in"=w365) -> ("error out"=w364:errorcluster)  [unwired: 8 in]
                }
                event "Exposure": Value Change {
                  n184 = event-data() -> ()  [unwired: 1 in, 1 out]
                  n185 = stacked-sequence {
                    tunnel: w371 -> [w374 _ w379 w382]
                    tunnel: [w372 _ _ _] -> w370
                    tunnel: w369 -> [_ _ _ _]
                    tunnel: w368 -> [_ w376 w378 _]
                    frame #0 {
                      n186 = property on="Exposure" class="DigNum (strict)"(error in=w374, "DisabledEnum"=T8."Disabled and Grayed Out" ("Disabled")) -> (error out=w372:errorcluster)  [unwired: 1 in, 1 out]
                    }
                    frame #1 {
                      n187 = call-dynamic "SetExposure.vi"("Exp"="Exposure", "camera.nit in"=w376) -> ()  [unwired: 9 in, 1 out]
                    }
                    frame #2 {
                      n188 = call "Stall Data Flow.vim"("value in"=w379, "milliseconds to wait"=u32 200) -> ()  [unwired: 2 out]
                      n189 = call "GetFPSrange.vi"("camera.nit_c in"=w378) -> ("current"=w377:dbl)  [unwired: 7 in, 3 out]
                      n190 = local write "FPS (For PL only)"(w377) -> ()
                    }
                    frame #3 {
                      n191 = property on="Exposure" class="DigNum (strict)"(error in=w382, "DisabledEnum"=T8."Enabled" ("Disabled")) -> ()  [unwired: 1 in, 2 out]
                    }
                  }
                }
                event "FPS (For PL only)": Value Change {
                  n192 = event-data() -> ()  [unwired: 1 in, 1 out]
                  n193 = stacked-sequence {
                    tunnel: w386 -> [w389 _ w393 w399]
                    tunnel: [w388 _ _ _] -> w385
                    tunnel: w384 -> [_ _ _ _]
                    tunnel: w383 -> [_ w391 w392 _]
                    frame #0 {
                      n194 = property on="FPS (For PL only)" class="DigNum (strict)"(error in=w389, "DisabledEnum"=T8."Disabled and Grayed Out" ("Disabled")) -> (error out=w388:errorcluster)  [unwired: 1 in, 1 out]
                    }
                    frame #1 {
                      n195 = call-dynamic "WriteFPS.vi"("FPS"="FPS (For PL only)", "camera.nit in"=w391) -> ()  [unwired: 9 in, 1 out]
                    }
                    frame #2 {
                      n196 = disable-structure shown="Disabled" {
                        disable-tunnel: w393 -> [w396 _]
                        disable-tunnel: w392 -> [w395 _]
                        frame Disabled {
                          n197 = call "Stall Data Flow.vim"("value in"=w396, "milliseconds to wait"=u32 200) -> ()  [unwired: 2 out]
                          n198 = call "GetFPSrange.vi"("camera.nit_c in"=w395) -> ("current"=w394:dbl)  [unwired: 7 in, 3 out]
                          n199 = local write "FPS (For PL only)"(w394) -> ()
                        }
                        frame Enabled {
                        }
                      }
                    }
                    frame #3 {
                      n200 = property on="FPS (For PL only)" class="DigNum (strict)"(error in=w399, "DisabledEnum"=T8."Enabled" ("Disabled")) -> ()  [unwired: 1 in, 2 out]
                    }
                  }
                }
                event "Gain": Value Change {
                  n201 = event-data() -> ()  [unwired: 1 in, 1 out]
                  n202 = call "SetGain.vi"("Gain"="Gain", "camera.nit in"=w402) -> ("error out"=w401:errorcluster)  [unwired: 9 in]
                }
                event "histogram.enable": Value Change {
                  n203 = event-data() -> ("NewVal"=w404:bool)  [unwired: 1 in]
                  n204 = call "conv.Disabled.vi"("NewVal"=w404) -> ("f"=w403:T8)  [unwired: 10 in]
                  n205 = property on="histogram" class="XYGraph (strict)"("DisabledEnum"=w403) -> ()  [unwired: 2 in, 2 out]
                  n206 = property on="# bins" class="DigNum (strict)"("DisabledEnum"=w403) -> ()  [unwired: 2 in, 2 out]
                }
                event "mapping", "Min Value", "Max Value": Value Change {
                  n207 = event-data() -> ()  [unwired: 1 in, 1 out]
                  n208 = case shown="4" "mapping" {
                    selector: "mapping" -> [w408 w411 w414]
                    frame Default {
                      n209 = property on="Image" class="ImageControl"("16-bit Display Conversion Method"=w408, "16-bit Display Maximum Value"="Max Value", "16-bit Display Minimum Value"="Min Value") -> ()  [unwired: 2 in, 2 out]
                    }
                    frame 6 {
                      n210 = property on="Image" class="ImageControl"("16-bit Display Conversion Method"=w411, "16-bit Display Maximum Value"=99 ("16-bit Display Mapping:Maximum Value"), "16-bit Display Minimum Value"=1 ("16-bit Display Mapping:Minimum Value")) -> ()  [unwired: 2 in, 2 out]
                    }
                    frame 4 {
                      n211 = property on="Image" class="ImageControl"("16-bit Display Conversion Method"=w414, "16-bit Display Maximum Value"=10000 ("16-bit Display Mapping:Maximum Value"), "16-bit Display Minimum Value"=0 ("16-bit Display Mapping:Minimum Value")) -> ()  [unwired: 2 in, 2 out]
                    }
                  }
                }
                event "state": Value Change {
                  n212 = event-data() -> ("NewVal"=w417:T2, "OldVal"=w415:T2)  [unwired: 1 in]
                  n213 = stacked-sequence {
                    tunnel: w419 -> [_ w426 _ _ w464 _]
                    tunnel: w418 -> [w422 _ w430 w445 w461 w472]
                    tunnel: w417 -> [_ _ w429 w439 w465 w473]
                    tunnel: w416 -> [_ _ w428 w444 _ _]
                    tunnel: w415 -> [_ _ _ w441 _ _]
                    frame #0 {
                      n214 = local write "video"(T3 FALSE ("video")) -> ()
                      n215 = property on="state" class="RadioBtnsControl (strict)"(error in=w422, "DisabledEnum"=T8."Disabled and Grayed Out" ("Disabled")) -> ()  [unwired: 1 in, 2 out]
                    }
                    frame #1 {
                      n216 = Unbundle By Name(w426) -> ("timing.state"=w425:refnum<queue>)
                      n217 = Flush Queue(queue=w425) -> (error out=w423:errorcluster)  [unwired: 1 in, 2 out]
                      n218 = call "Stall Data Flow.vim"("value in"=w423, "milliseconds to wait"=u32 150) -> ()  [unwired: 2 out]
                    }
                    frame #2 {
                      n219 = call "Stall Data Flow.vim"("value in"=w430, "milliseconds to wait"=u32 150) -> ("value out"=w427:errorcluster)  [unwired: 1 out]
                      n220 = case shown="\"Switch\"" w429 {
                        tunnel: w428 -> [_ w433]
                        tunnel: w427 -> [_ w432]
                        frame Default {
                        }
                        frame "Switch" {
                          n221 = local read "FPS (For PL only)"() -> (w434:dbl)
                          n222 = call-dynamic "WriteFPS.vi"("error in"=w432, "FPS"=w434, "camera.nit in"=w433) -> ()  [unwired: 8 in, 1 out]
                        }
                      }
                    }
                    frame #3 {
                      n223 = Equal?(x=T2."Single", y=w439) -> (x = y?=w436:bool)
                      n224 = Equal?(x=w441, y=T2."none") -> (x = y?=w437:bool)
                      n225 = And(x=w436, y=w437) -> (x .and. y?=w435:bool)
                      n226 = case shown="\"none\"" w439 {
                        tunnel: [w450 w452 w454 w456 w458 w460] -> w443
                        tunnel: [T8."Disabled and Grayed Out" ("Disabled") T8."Disabled and Grayed Out" ("Disabled") T8."Disabled and Grayed Out" ("Disabled") T8."Enabled" ("Disabled") T8."Enabled" ("Disabled") T8."Disabled and Grayed Out" ("Disabled")] -> w442
                        frame Default {
                          w450 = T13 0 items=["none", "IR", "LivePL", "PL"] ("DLL.state")
                        }
                        frame "Switch" {
                          w452 = T13 3 items=["none", "IR", "LivePL", "PL"] ("DLL.state")
                        }
                        frame "Single" {
                          w454 = T13 1 items=["none", "IR", "LivePL", "PL"] ("DLL.state")
                        }
                        frame "Video" {
                          w456 = T13 1 items=["none", "IR", "LivePL", "PL"] ("DLL.state")
                        }
                        frame "Live" {
                          w458 = T13 2 items=["none", "IR", "LivePL", "PL"] ("DLL.state")
                        }
                        frame "none" {
                          w460 = T13 0 items=["none", "IR", "LivePL", "PL"] ("DLL.state")
                        }
                      }
                      n227 = case shown="False" w435 {
                        tunnel: w445 -> [w448 _]
                        tunnel: w444 -> [w447 _]
                        tunnel: w443 -> [w446 _]
                        frame False {
                          n228 = call "SetState.vi"("error in"=w448, "DLL.state"=w446, "camera in"=w447) -> ()  [unwired: 8 in, 1 out]
                        }
                        frame True {
                        }
                      }
                      n229 = property on="Exposure" class="DigNum (strict)"("DisabledEnum"=w442) -> ()  [unwired: 2 in, 2 out]
                      n230 = property on="video" class="Bool (strict)"("DisabledEnum"=w442) -> ()  [unwired: 2 in, 2 out]
                    }
                    frame #4 {
                      n231 = Unbundle By Name(w464) -> ("timing.state"=w463:refnum<queue>)
                      n232 = case shown="\"Video\"" w465 {
                        tunnel: [state."-" ("element") state."PL" ("element") state."single" ("element") state."video" ("element") state."livePL" ("element") state."-" ("element")] -> w462
                        frame Default {
                        }
                        frame "Switch" {
                        }
                        frame "Single" {
                        }
                        frame "Video" {
                        }
                        frame "Live" {
                        }
                        frame "none" {
                        }
                      }
                      n233 = Lossy Enqueue Element(queue=w463, element=w462, error in (no error)=w461) -> ()  [unwired: 4 out]
                    }
                    frame #5 {
                      n234 = case shown="\"Single\"..\"Live\"" w473 {
                        tunnel: w472 -> [_ w476]
                        frame Default {
                        }
                        frame "Single".."Live" {
                          n235 = call "Stall Data Flow.vim"("value in"=w476, "milliseconds to wait"=u32 250) -> ("value out"=w475:errorcluster)  [unwired: 1 out]
                          n236 = local write "progress"(u8 0 ("progress")) -> ()
                          n237 = property on="state" class="RadioBtnsControl (strict)"(error in=w475, "DisabledEnum"=T8."Enabled" ("Disabled")) -> ()  [unwired: 1 in, 2 out]
                        }
                      }
                    }
                  }
                }
                event "Module Name": Mouse Up {
                  n238 = event-data() -> ()  [unwired: 1 in, 1 out]
                  n239 = call "keyboard.vi"() -> ()  [unwired: 12 in]
                }
                event "Exposure", "Acquisitions": Mouse Up {
                  n240 = event-data() -> ("Coords.Horizontal"=w481:i32)  [unwired: 1 in]
                  n241 = call "sem.Acquire.vi"("camera.nit in"=w479) -> ()  [unwired: 10 in, 1 out]
                  n242 = in-place {
                    in-place-border: w481 -> [w483]
                    in-place-border: w479 -> [w482]
                    in-place-border: [w482] -> w480
                    n243 = property on="Exposure" class="DigNum (strict)"() -> ("Width"=w485:u32, "Left"=w484:i32)  [unwired: 2 in, 2 out]
                    n244 = call "clickableRange.vi"("Horizontal"=w483, "Left"=w484, "Width"=w485) -> ()  [unwired: 9 in]
                  }
                  n245 = call "sem.Release.vi"("camera.nit in"=w480) -> ()  [unwired: 10 in, 1 out]
                }
                event "Acquisitions": Value Change {
                  n246 = event-data() -> ()  [unwired: 1 in, 1 out]
                  n247 = call "SetAcquisitions.vi"("error in"=w491, "Acquisitions"="Acquisitions", "camera in"=w490) -> ("error out"=w487:errorcluster)  [unwired: 8 in]
                  n248 = call "DVR.number_acq.Write.vi"("error in"=w487, "# acq"="Acquisitions", "DVR in"=w489) -> ("error out"=w486:errorcluster)  [unwired: 8 in]
                }
                event "plus": Value Change {
                  w494 = u32 9 items=["Zoom Tool"=8, "Selection Tool"=0, "Pan Tool"=9, "Point Tool"=1, "Line Tool"=2, "Rectangle Tool"=3, "Rotated Rectangle Tool"=12, "Polyline Tool"=10, "Polygon Tool"=5, "Freehand Tool"=11, "Closed Freehand Tool"=6, "Ellipse Tool"=4, "Annulus Tool"=7] ("Current ROI Tool")
                  n249 = event-data() -> ()  [unwired: 1 in, 1 out]
                  n250 = property on="Image" class="ImageControl"(error in=w497) -> (error out=w496:errorcluster, "ZoomSingle"=w499:cluster{"X":sgl, "Y":sgl})  [unwired: 1 in, 1 out]
                  n251 = Multiply(x=w499, y=1.2) -> (x*y=w495:cluster{"X":dbl, "Y":dbl})
                  n252 = property on="Image" class="ImageControl"(error in=w496, "ZoomSingle"=w495) -> (error out=w493:errorcluster)  [unwired: 1 in, 1 out]
                  n253 = property on="Image" class="ImageControl"(error in=w493, "Current ROI Tool"=w494) -> (error out=w492:errorcluster)  [unwired: 1 in, 1 out]
                }
                event "minus": Value Change {
                  w502 = u32 9 items=["Zoom Tool"=8, "Selection Tool"=0, "Pan Tool"=9, "Point Tool"=1, "Line Tool"=2, "Rectangle Tool"=3, "Rotated Rectangle Tool"=12, "Polyline Tool"=10, "Polygon Tool"=5, "Freehand Tool"=11, "Closed Freehand Tool"=6, "Ellipse Tool"=4, "Annulus Tool"=7] ("Current ROI Tool")
                  n254 = event-data() -> ()  [unwired: 1 in, 1 out]
                  n255 = property on="Image" class="ImageControl"(error in=w505) -> (error out=w504:errorcluster, "ZoomSingle"=w507:cluster{"X":sgl, "Y":sgl})  [unwired: 1 in, 1 out]
                  n256 = Divide(x=w507, y=1.2) -> (x/y=w503:cluster{"X":dbl, "Y":dbl})
                  n257 = property on="Image" class="ImageControl"(error in=w504, "ZoomSingle"=w503) -> (error out=w501:errorcluster)  [unwired: 1 in, 1 out]
                  n258 = property on="Image" class="ImageControl"(error in=w501, "Current ROI Tool"=w502) -> (error out=w500:errorcluster)  [unwired: 1 in, 1 out]
                }
                event "fit": Value Change {
                  n259 = event-data() -> ()  [unwired: 1 in, 1 out]
                  n260 = property on="Image" class="ImageControl"(error in=w509, "Zoom to Fit Mode"=TRUE) -> (error out=w510:errorcluster)  [unwired: 1 in, 1 out]
                }
              }
            }
            frame Error {
              n261 = call <vilib>:"Simple Error Handler.vi"("error in (no error)"=w511) -> ()  [unwired: 4 in, 5 out]
            }
          }
        }
        n262 = call-dynamic "Run.vi"("camera.nit in"=w221) -> ()  [unwired: 10 in, 1 out]
        n263 = Merge Errors(w226, w224) -> (w225:errorcluster)
      }
      frame Default {
        # "Done!"
        n264 = Unbundle By Name(w514) -> ("ref.rightPanel"=w523:refnum<vi>)
        n265 = property class="TabCtl (strict)"(reference=w523, "DisabledEnum"=T8."Enabled" ("Disabled")) -> ()  [unwired: 1 in, 2 out]
        n266 = Unbundle By Name(w514) -> ("ref.graph.avi"=w517:T1, "ref.graph.img"=w518:T1, "timing.closeLoop"=w520:refnum<notifier>, "timing.state"=w521:refnum<queue>, "cam"=w513:refnum<class "camera.lvclass">)
        n267 = call-dynamic "Uninit.vi"("error in"=w512, "camera.nit in"=w513) -> ("error out"=w519:errorcluster)  [unwired: 9 in]
        n268 = disable-structure shown="Disabled" {
          frame Disabled {
            n269 = call "histogram.vi"("# bins"="# bins") -> ("histogram"=→"histogram":cluster{"Axis":dbl[], "Histogram":i32[]})  [unwired: 10 in]
          }
          frame Enabled {
          }
        }
        n270 = Release Queue(queue=w521) -> ()  [unwired: 2 in, 3 out]
        n271 = Release Notifier(notifier=w520) -> ()  [unwired: 2 in, 3 out]
        n272 = call "IMAQ Dispose"("Image"=w518) -> ()  [unwired: 5 in, 1 out]
        n273 = call "IMAQ Dispose"("Image"=w517) -> ()  [unwired: 5 in, 1 out]
        n274 = call "Stall Data Flow.vim"("value in"=w519, "milliseconds to wait"=u32 1000) -> ("value out"=w516:errorcluster)  [unwired: 1 out]
      }
    }
  }
  n275 = disable-structure shown="RUN_TIME_ENGINE==True" {
    disable-tunnel: w3 -> [_ _]
    frame condition #0 {
      n276 = Quit LabVIEW(quit? (T)=TRUE) -> ()
    }
    frame condition #1 (active) {
    }
  }
